vi "GetProbePlanCoordinates.vi"(8 "Use index as X coord":bool=TRUE, 9 "Probe Card Channels":i32=1) -> (0 "file path":string, 2 "OK?":bool, 3 "Array":T1(array[cluster]))   [LabVIEW 2018] (continued)
863\tX=17755.26\ty=25056.33 \nLabel=Strip\t864\tX=18099.17\ty=25163.49 \nLabel=Strip\t865\tX=17745.54\ty=25211.79 \nLabel=Strip\t866\tX=18089.41\ty=25319.09 \nLabel=Strip\t867\tX=17735.76\ty=25367.26 \nLabel=Strip\t868\tX=18079.58\ty=25474.68 \nLabel=Strip\t869\tX=17725.92\ty=25522.72 \nLabel=Strip\t870\tX=18069.70\ty=25630.28 \nLabel=Strip\t871\tX=17716.01\ty=25678.17 \nLabel=Strip\t872\tX=18059.75\ty=25785.87 \nLabel=Strip\t873\tX=17706.05\ty=25833.63 \nLabel=Strip\t874\tX=18049.75\ty=25941.46 \nLabel=Strip\t875\tX=17696.03\ty=25989.08 \nLabel=Strip\t876\tX=18039.68\ty=26097.04 \nLabel=Strip\t877\tX=17685.94\ty=26144.53 \nLabel=Strip\t878\tX=18029.56\ty=26252.63 \nLabel=Strip\t879\tX=17675.80\ty=26299.98 \nLabel=Strip\t880\tX=18019.37\ty=26408.21 \nLabel=Strip\t881\tX=17665.59\ty=26455.42 \nLabel=Strip\t882\tX=18009.13\ty=26563.79 \nLabel=Strip\t883\tX=17655.33\ty=26610.87 \nLabel=Strip\t884\tX=17998.82\ty=26719.39 \nLabel=Strip\t885\tX=17645.01\ty=26766.31 \nLabel=Strip\t886\tX=17988.45\ty=26874.93 \nLabel=Strip\t887\tX=17634.62\ty=26921.74 \nLabel=Strip\t888\tX=17978.03\ty=27030.50 \nLabel=Strip\t889\tX=17624.18\ty=27077.18 \nLabel=Strip\t890\tX=17967.54\ty=27186.07 \nLabel=Strip\t891\tX=17613.67\ty=27232.61 \nLabel=Strip\t892\tX=17956.99\ty=27341.64 \nLabel=Strip\t893\tX=17603.11\ty=27388.04 \nLabel=Strip\t894\tX=17946.37\ty=27497.34 \nLabel=Strip\t895\tX=17592.48\ty=27543.46 \nLabel=Strip\t896\tX=17935.72\ty=27652.76 \nLabel=Strip\t897\tX=17581.80\ty=27698.89 \nLabel=Strip\t898\tX=17924.99\ty=27808.31 \nLabel=Strip\t899\tX=17571.05\ty=27854.31 \nLabel=Strip\t900\tX=17914.20\ty=27963.87 \nLabel=Strip\t901\tX=17560.24\ty=28009.72 \nLabel=Strip\t902\tX=17903.35\ty=28119.42 \nLabel=Strip\t903\tX=17549.38\ty=28165.14 \nLabel=Strip\t904\tX=17892.45\ty=28274.96 \nLabel=Strip\t905\tX=17538.45\ty=28320.55 \nLabel=Strip\t906\tX=17881.48\ty=28430.51 \nLabel=Strip\t907\tX=17527.46\ty=28475.96 \nLabel=Strip\t908\tX=17870.45\ty=28586.05 \nLabel=Strip\t909\tX=17516.42\ty=28631.36 \nLabel=Strip\t910\tX=17859.36\ty=28741.59 \nLabel=Strip\t911\tX=17505.31\ty=28786.77 \nLabel=Strip\t912\tX=17848.21\ty=28897.13 \nLabel=Strip\t913\tX=17494.14\ty=28942.17 \nLabel=Strip\t914\tX=17837.00\ty=29052.66 \nLabel=Strip\t915\tX=17482.92\ty=29097.56 \nLabel=Strip\t916\tX=17825.73\ty=29208.19 \nLabel=Strip\t917\tX=17471.63\ty=29252.96 \nLabel=Strip\t918\tX=17814.40\ty=29363.71 \nLabel=Strip\t919\tX=17460.28\ty=29408.35 \nLabel=Strip\t920\tX=17803.00\ty=29519.24 \nLabel=Strip\t921\tX=17448.87\ty=29563.73 \nLabel=Strip\t922\tX=17791.55\ty=29674.76 \nLabel=Strip\t923\tX=17437.40\ty=29719.12 \nLabel=Strip\t924\tX=17780.04\ty=29830.28 \nLabel=Strip\t925\tX=17425.87\ty=29874.50 \nLabel=Strip\t926\tX=17768.47\ty=29985.79 \nLabel=Strip\t927\tX=17414.28\ty=30029.88 \nLabel=Strip\t928\tX=17756.84\ty=30141.30 \nLabel=Strip\t929\tX=17402.63\ty=30185.25 \nLabel=Strip\t930\tX=17745.15\ty=30296.81 \nLabel=Strip\t931\tX=17390.93\ty=30340.62 \nLabel=Strip\t932\tX=17733.39\ty=30452.31 \nLabel=Strip\t933\tX=17379.16\ty=30495.99 \nLabel=Strip\t934\tX=17721.58\ty=30607.81 \nLabel=Strip\t935\tX=17367.33\ty=30651.36 \nLabel=Strip\t936\tX=17709.71\ty=30763.31 \nLabel=Strip\t937\tX=17355.44\ty=30806.72 \nLabel=Strip\t938\tX=17697.77\ty=30918.81 \nLabel=Strip\t939\tX=17343.49\ty=30962.08 \nLabel=Strip\t940\tX=17685.78\ty=31074.30 \nLabel=Strip\t941\tX=17331.48\ty=31117.43 \nLabel=Strip\t942\tX=17673.73\ty=31229.79 \nLabel=Strip\t943\tX=17319.41\ty=31272.78 \nLabel=Strip\t944\tX=17661.61\ty=31385.27 \nLabel=Strip\t945\tX=17307.27\ty=31428.13 \nLabel=Strip\t946\tX=17649.44\ty=31540.75 \nLabel=Strip\t947\tX=17295.08\ty=31583.48 \nLabel=Strip\t948\tX=17637.20\ty=31696.23 \nLabel=Strip\t949\tX=17282.83\ty=31738.82 \nLabel=Strip\t950\tX=17624.91\ty=31851.70 \nLabel=Strip\t951\tX=17270.52\ty=31894.16 \nLabel=Strip\t952\tX=17612.55\ty=32007.17 \nLabel=Strip\t953\tX=17258.15\ty=32049.49 \nLabel=Strip\t954\tX=17600.14\ty=32162.64 \nLabel=Strip\t955\tX=17245.72\ty=32204.82 \nLabel=Strip\t956\tX=17587.66\ty=32318.10 \nLabel=Strip\t957\tX=17233.22\ty=32360.15 \nLabel=Strip\t958\tX=17575.13\ty=32473.56 \nLabel=Strip\t959\tX=17220.67\ty=32515.47 \nLabel=Strip\t960\tX=17562.53\ty=32629.02 \nLabel=Strip\t961\tX=17208.06\ty=32670.79 \nLabel=Strip\t962\tX=17549.87\ty=32784.47 \nLabel=Strip\t963\tX=17195.39\ty=32826.11 \nLabel=Strip\t964\tX=17537.16\ty=32939.92 \nLabel=Strip\t965\tX=17182.65\ty=32981.42 \nLabel=Strip\t966\tX=17524.38\ty=33095.37 \nLabel=Strip\t967\tX=17169.86\ty=33136.73 \nLabel=Strip\t968\tX=17511.54\ty=33250.81 \nLabel=Strip\t969\tX=17157.01\ty=33292.04 \nLabel=Strip\t970\tX=17498.64\ty=33406.25 \nLabel=Strip\t971\tX=17144.09\ty=33447.34 \nLabel=Strip\t972\tX=17485.69\ty=33561.68 \nLabel=Strip\t973\tX=17131.12\ty=33602.64 \nLabel=Strip\t974\tX=17472.67\ty=33717.12 \nLabel=Strip\t975\tX=17118.09\ty=33757.93 \nLabel=Strip\t976\tX=17459.59\ty=33872.54 \nLabel=Strip\t977\tX=17104.99\ty=33913.23 \nLabel=Strip\t978\tX=17446.45\ty=34027.97 \nLabel=Strip\t979\tX=17091.84\ty=34068.51 \nLabel=Strip\t980\tX=17433.25\ty=34183.39 \nLabel=Strip\t981\tX=17078.62\ty=34223.80 \nLabel=Strip\t982\tX=17419.99\ty=34338.80 \nLabel=Strip\t983\tX=17065.35\ty=34379.08 \nLabel=Strip\t984\tX=17406.67\ty=34494.21 \nLabel=Strip\t985\tX=17052.01\ty=34534.35 \nLabel=Strip\t986\tX=17393.29\ty=34649.62 \nLabel=Strip\t987\tX=17038.62\ty=34689.62 \nLabel=Strip\t988\tX=17379.85\ty=34805.03 \nLabel=Strip\t989\tX=17025.16\ty=34844.89 \nLabel=Strip\t990\tX=17366.35\ty=34960.43 \nLabel=Strip\t991\tX=17011.65\ty=35000.16 \nLabel=Strip\t992\tX=17352.79\ty=35115.82 \nLabel=Strip\t993\tX=16998.07\ty=35155.42 \nLabel=Strip\t994\tX=17339.17\ty=35271.21 \nLabel=Strip\t995\tX=16984.43\ty=35310.67 \nLabel=Strip\t996\tX=17325.49\ty=35426.60 \nLabel=Strip\t997\tX=16970.74\ty=35465.92 \nLabel=Strip\t998\tX=17311.75\ty=35581.99 \nLabel=Strip\t999\tX=16956.98\ty=35621.17 \nLabel=Strip\t1000\tX=17297.95\ty=35737.37 \nLabel=Strip\t1001\tX=16943.16\ty=35776.42 \nLabel=Strip\t1002\tX=17284.09\ty=35892.74 \nLabel=Strip\t1003\tX=16929.29\ty=35931.66 \nLabel=Strip\t1004\tX=17270.17\ty=36048.12 \nLabel=Strip\t1005\tX=16915.35\ty=36086.89 \nLabel=Strip\t1006\tX=17256.18\ty=36203.49 \nLabel=Strip\t1007\tX=16901.35\ty=36242.12 \nLabel=Strip\t1008\tX=17242.14\ty=36358.85 \nLabel=Strip\t1009\tX=16887.30\ty=36397.35 \nLabel=Strip\t1010\tX=17228.04\ty=36514.21 \nLabel=Strip\t1011\tX=16873.18\ty=36552.57 \nLabel=Strip\t1012\tX=17213.87\ty=36669.56 \nLabel=Strip\t1013\tX=16859.00\ty=36707.79 \nLabel=Strip\t1014\tX=17199.65\ty=36824.92 \nLabel=Strip\t1015\tX=16844.76\ty=36863.01 \nLabel=Strip\t1016\tX=17185.37\ty=36980.26 \nLabel=Strip\t1017\tX=16830.46\ty=37018.22 \nLabel=Strip\t1018\tX=17171.03\ty=37135.61 \nLabel=Strip\t1019\tX=16816.11\ty=37173.43 \nLabel=Strip\t1020\tX=17156.62\ty=37290.95 \nLabel=Strip\t1021\tX=16801.69\ty=37328.63 \nLabel=Strip\t1022\tX=17142.16\ty=37446.28 \nLabel=Strip\t1023\tX=16787.21\ty=37483.83 \nLabel=Strip\t1024\tX=17127.63\ty=37601.61 \nLabel=Strip\t1025\tX=16772.67\ty=37639.02 \nLabel=Strip\t1026\tX=17113.05\ty=37756.94 \nRegion=Segment\t2B\nLabel=Strip\t1\tX=17590.21\ty=-41968.68 \nLabel=Strip\t2\tX=17947.11\ty=-41920.02 \nLabel=Strip\t3\tX=17606.36\ty=-41813.84 \nLabel=Strip\t4\tX=17963.24\ty=-41765.04 \nLabel=Strip\t5\tX=17622.45\ty=-41658.99 \nLabel=Strip\t6\tX=17979.31\ty=-41610.05 \nLabel=Strip\t7\tX=17638.47\ty=-41504.13 \nLabel=Strip\t8\tX=17995.31\ty=-41455.05 \nLabel=Strip\t9\tX=17654.44\ty=-41349.26 \nLabel=Strip\t10\tX=18011.26\ty=-41300.04 \nLabel=Strip\t11\tX=17670.35\ty=-41194.38 \nLabel=Strip\t12\tX=18027.15\ty=-41145.03 \nLabel=Strip\t13\tX=17686.20\ty=-41039.50 \nLabel=Strip\t14\tX=18042.98\ty=-40990.01 \nLabel=Strip\t15\tX=17701.99\ty=-40884.61 \nLabel=Strip\t16\tX=18058.75\ty=-40834.98 \nLabel=Strip\t17\tX=17717.72\ty=-40729.71 \nLabel=Strip\t18\tX=18074.46\ty=-40679.94 \nLabel=Strip\t19\tX=17733.38\ty=-40574.81 \nLabel=Strip\t20\tX=18090.11\ty=-40524.90 \nLabel=Strip\t21\tX=17748.99\ty=-40419.89 \nLabel=Strip\t22\tX=18105.70\ty=-40369.85 \nLabel=Strip\t23\tX=17764.54\ty=-40264.98 \nLabel=Strip\t24\tX=18121.23\ty=-40214.79 \nLabel=Strip\t25\tX=17780.04\ty=-40110.05 \nLabel=Strip\t26\tX=18136.71\ty=-40059.73 \nLabel=Strip\t27\tX=17795.47\ty=-39955.11 \nLabel=Strip\t28\tX=18152.12\ty=-39904.65 \nLabel=Strip\t29\tX=17810.84\ty=-39800.17 \nLabel=Strip\t30\tX=18167.47\ty=-39749.57 \nLabel=Strip\t31\tX=17826.15\ty=-39645.22 \nLabel=Strip\t32\tX=18182.76\ty=-39594.49 \nLabel=Strip\t33\tX=17841.40\ty=-39490.27 \nLabel=Strip\t34\tX=18197.99\ty=-39439.39 \nLabel=Strip\t35\tX=17856.60\ty=-39335.31 \nLabel=Strip\t36\tX=18213.17\ty=-39284.29 \nLabel=Strip\t37\tX=17871.73\ty=-39180.34 \nLabel=Strip\t38\tX=18228.28\ty=-39129.18 \nLabel=Strip\t39\tX=17886.80\ty=-39025.36 \nLabel=Strip\t40\tX=18243.34\ty=-38974.07 \nLabel=Strip\t41\tX=17901.82\ty=-38870.38 \nLabel=Strip\t42\tX=18258.33\ty=-38818.95 \nLabel=Strip\t43\tX=17916.77\ty=-38715.38 \nLabel=Strip\t44\tX=18273.27\ty=-38663.82 \nLabel=Strip\t45\tX=17931.67\ty=-38560.39 \nLabel=Strip\t46\tX=18288.14\ty=-38508.68 \nLabel=Strip\t47\tX=17946.50\ty=-38405.38 \nLabel=Strip\t48\tX=18302.96\ty=-38353.54 \nLabel=Strip\t49\tX=17961.28\ty=-38250.37 \nLabel=Strip\t50\tX=18317.71\ty=-38198.39 \nLabel=Strip\t51\tX=17975.99\ty=-38095.35 \nLabel=Strip\t52\tX=18332.41\ty=-38043.23 \nLabel=Strip\t53\tX=17990.65\ty=-37940.32 \nLabel=Strip\t54\tX=18347.04\ty=-37888.06 \nLabel=Strip\t55\tX=18005.25\ty=-37785.29 \nLabel=Strip\t56\tX=18361.62\ty=-37732.89 \nLabel=Strip\t57\tX=18019.78\ty=-37630.25 \nLabel=Strip\t58\tX=18376.14\ty=-37577.71 \nLabel=Strip\t59\tX=18034.26\ty=-37475.20 \nLabel=Strip\t60\tX=18390.59\ty=-37422.53 \nLabel=Strip\t61\tX=18048.68\ty=-37320.15 \nLabel=Strip\t62\tX=18404.99\ty=-37267.34 \nLabel=Strip\t63\tX=18063.04\ty=-37165.09 \nLabel=Strip\t64\tX=18419.33\ty=-37112.14 \nLabel=Strip\t65\tX=18077.33\ty=-37010.02 \nLabel=Strip\t66\tX=18433.61\ty=-36956.93 \nLabel=Strip\t67\tX=18091.57\ty=-36854.95 \nLabel=Strip\t68\tX=18447.83\ty=-36801.72 \nLabel=Strip\t69\tX=18105.75\ty=-36699.86 \nLabel=Strip\t70\tX=18461.98\ty=-36646.50 \nLabel=Strip\t71\tX=18119.87\ty=-36544.78 \nLabel=Strip\t72\tX=18476.08\ty=-36491.27 \nLabel=Strip\t73\tX=18133.93\ty=-36389.68 \nLabel=Strip\t74\tX=18490.12\ty=-36336.04 \nLabel=Strip\t75\tX=18147.93\ty=-36234.58 \nLabel=Strip\t76\tX=18504.10\ty=-36180.80 \nLabel=Strip\t77\tX=18161.87\ty=-36079.47 \nLabel=Strip\t78\tX=18518.02\ty=-36025.55 \nLabel=Strip\t79\tX=18175.75\ty=-35924.36 \nLabel=Strip\t80\tX=18531.88\ty=-35870.30 \nLabel=Strip\t81\tX=18189.57\ty=-35769.24 \nLabel=Strip\t82\tX=18545.68\ty=-35715.04 \nLabel=Strip\t83\tX=18203.33\ty=-35614.11 \nLabel=Strip\t84\tX=18559.42\ty=-35559.78 \nLabel=Strip\t85\tX=18217.04\ty=-35458.97 \nLabel=Strip\t86\tX=18573.10\ty=-35404.50 \nLabel=Strip\t87\tX=18230.68\ty=-35303.83 \nLabel=Strip\t88\tX=18586.72\ty=-35249.22 \nLabel=Strip\t89\tX=18244.26\ty=-35148.69 \nLabel=Strip\t90\tX=18600.28\ty=-35093.94 \nLabel=Strip\t91\tX=18257.78\ty=-34993.53 \nLabel=Strip\t92\tX=18613.78\ty=-34938.65 \nLabel=Strip\t93\tX=18271.25\ty=-34838.37 \nLabel=Strip\t94\tX=18627.23\ty=-34783.35 \nLabel=Strip\t95\tX=18284.65\ty=-34683.20 \nLabel=Strip\t96\tX=18640.61\ty=-34628.04 \nLabel=Strip\t97\tX=18297.99\ty=-34528.03 \nLabel=Strip\t98\tX=18653.93\ty=-34472.73 \nLabel=Strip\t99\tX=18311.28\ty=-34372.85 \nLabel=Strip\t100\tX=18667.19\ty=-34317.41 \nLabel=Strip\t101\tX=18324.50\ty=-34217.66 \nLabel=Strip\t102\tX=18680.40\ty=-34162.09 \nLabel=Strip\t103\tX=18337.66\ty=-34062.47 \nLabel=Strip\t104\tX=18693.54\ty=-34006.76 \nLabel=Strip\t105\tX=18350.77\ty=-33907.27 \nLabel=Strip\t106\tX=18706.62\ty=-33851.42 \nLabel=Strip\t107\tX=18363.81\ty=-33752.06 \nLabel=Strip\t108\tX=18719.64\ty=-33696.08 \nLabel=Strip\t109\tX=18376.80\ty=-33596.85 \nLabel=Strip\t110\tX=18732.61\ty=-33540.73 \nLabel=Strip\t111\tX=18389.72\ty=-33441.64 \nLabel=Strip\t112\tX=18745.51\ty=-33385.37 \nLabel=Strip\t113\tX=18402.59\ty=-33286.41 \nLabel=Strip\t114\tX=18758.35\ty=-33230.01 \nLabel=Strip\t115\tX=18415.39\ty=-33131.18 \nLabel=Strip\t116\tX=18771.14\ty=-33074.64 \nLabel=Strip\t117\tX=18428.14\ty=-32975.94 \nLabel=Strip\t118\tX=18783.86\ty=-32919.26 \nLabel=Strip\t119\tX=18440.83\ty=-32820.70 \nLabel=Strip\t120\tX=18796.53\ty=-32763.88 \nLabel=Strip\t121\tX=18453.45\ty=-32665.45 \nLabel=Strip\t122\tX=18809.13\ty=-32608.49 \nLabel=Strip\t123\tX=18466.02\ty=-32510.19 \nLabel=Strip\t124\tX=18821.68\ty=-32453.10 \nLabel=Strip\t125\tX=18478.53\ty=-32354.93 \nLabel=Strip\t126\tX=18834.16\ty=-32297.70 \nLabel=Strip\t127\tX=18490.97\ty=-32199.67 \nLabel=Strip\t128\tX=18846.59\ty=-32142.30 \nLabel=Strip\t129\tX=18503.36\ty=-32044.39 \nLabel=Strip\t130\tX=18858.95\ty=-31986.88 \nLabel=Strip\t131\tX=18515.69\ty=-31889.11 \nLabel=Strip\t132\tX=18871.26\ty=-31831.47 \nLabel=Strip\t133\tX=18527.96\ty=-31733.83 \nLabel=Strip\t134\tX=18883.50\ty=-31676.04 \nLabel=Strip\t135\tX=18540.16\ty=-31578.53 \nLabel=Strip\t136\tX=18895.69\ty=-31520.61 \nLabel=Strip\t137\tX=18552.31\ty=-31423.24 \nLabel=Strip\t138\tX=18907.81\ty=-31365.18 \nLabel=Strip\t139\tX=18564.40\ty=-31267.93 \nLabel=Strip\t140\tX=18919.88\ty=-31209.73 \nLabel=Strip\t141\tX=18576.43\ty=-31112.62 \nLabel=Strip\t142\tX=18931.89\ty=-31054.29 \nLabel=Strip\t143\tX=18588.40\ty=-30957.31 \nLabel=Strip\t144\tX=18943.83\ty=-30898.83 \nLabel=Strip\t145\tX=18600.31\ty=-30801.99 \nLabel=Strip\t146\tX=18955.72\ty=-30743.37 \nLabel=Strip\t147\tX=18612.16\ty=-30646.66 \nLabel=Strip\t148\tX=18967.55\ty=-30587.91 \nLabel=Strip\t149\tX=18623.94\ty=-30491.32 \nLabel=Strip\t150\tX=18979.31\ty=-30432.44 \nLabel=Strip\t151\tX=18635.67\ty=-30335.98 \nLabel=Strip\t152\tX=18991.02\ty=-30276.96 \nLabel=Strip\t153\tX=18647.34\ty=-30180.64 \nLabel=Strip\t154\tX=19002.67\ty=-30121.48 \nLabel=Strip\t155\tX=18658.95\ty=-30025.29 \nLabel=Strip\t156\tX=19014.25\ty=-29965.99 \nLabel=Strip\t157\tX=18670.50\ty=-29869.93 \nLabel=Strip\t158\tX=19025.78\ty=-29810.49 \nLabel=Strip\t159\tX=18682.00\ty=-29714.57 \nLabel=Strip\t160\tX=19037.25\ty=-29654.99 \nLabel=Strip\t161\tX=18693.43\ty=-29559.20 \nLabel=Strip\t162\tX=19048.66\ty=-29499.49 \nLabel=Strip\t163\tX=18704.80\ty=-29403.83 \nLabel=Strip\t164\tX=19060.00\ty=-29343.98 \nLabel=Strip\t165\tX=18716.11\ty=-29248.45 \nLabel=Strip\t166\tX=19071.29\ty=-29188.46 \nLabel=Strip\t167\tX=18727.36\ty=-29093.06 \nLabel=Strip\t168\tX=19082.52\ty=-29032.93 \nLabel=Strip\t169\tX=18738.55\ty=-28937.67 \nLabel=Strip\t170\tX=19093.69\ty=-28877.41 \nLabel=Strip\t171\tX=18749.68\ty=-28782.28 \nLabel=Strip\t172\tX=19104.80\ty=-28721.87 \nLabel=Strip\t173\tX=18760.75\ty=-28626.87 \nLabel=Strip\t174\tX=19115.84\ty=-28566.33 \nLabel=Strip\t175\tX=18771.76\ty=-28471.47 \nLabel=Strip\t176\tX=19126.83\ty=-28410.79 \nLabel=Strip\t177\tX=18782.72\ty=-28316.05 \nLabel=Strip\t178\tX=19137.76\ty=-28255.24 \nLabel=Strip\t179\tX=18793.61\ty=-28160.63 \nLabel=Strip\t180\tX=19148.63\ty=-28099.68 \nLabel=Strip\t181\tX=18804.44\ty=-28005.21 \nLabel=Strip\t182\tX=19159.44\ty=-27944.12 \nLabel=Strip\t183\tX=18815.21\ty=-27849.78 \nLabel=Strip\t184\tX=19170.19\ty=-27788.55 \nLabel=Strip\t185\tX=18825.92\ty=-27694.35 \nLabel=Strip\t186\tX=19180.88\ty=-27632.98 \nLabel=Strip\t187\tX=18836.58\ty=-27538.90 \nLabel=Strip\t188\tX=19191.50\ty=-27477.40 \nLabel=Strip\t189\tX=18847.17\ty=-27383.46 \nLabel=Strip\t190\tX=19202.07\ty=-27321.82 \nLabel=Strip\t191\tX=18857.70\ty=-27228.01 \nLabel=Strip\t192\tX=19212.58\ty=-27166.23 \nLabel=Strip\t193\tX=18868.17\ty=-27072.55 \nLabel=Strip\t194\tX=19223.03\ty=-27010.63 \nLabel=Strip\t195\tX=18878.59\ty=-26917.09 \nLabel=Strip\t196\tX=19233.42\ty=-26855.03 \nLabel=Strip\t197\tX=18888.94\ty=-26761.62 \nLabel=Strip\t198\tX=19243.75\ty=-26699.43 \nLabel=Strip\t199\tX=18899.23\ty=-26606.15 \nLabel=Strip\t200\tX=19254.02\ty=-26543.82 \nLabel=Strip\t201\tX=18909.47\ty=-26450.67 \nLabel=Strip\t202\tX=19264.23\ty=-26388.20 \nLabel=Strip\t203\tX=18919.64\ty=-26295.19 \nLabel=Strip\t204\tX=19274.38\ty=-26232.58 \nLabel=Strip\t205\tX=18929.75\ty=-26139.70 \nLabel=Strip\t206\tX=19284.47\ty=-26076.96 \nLabel=Strip\t207\tX=18939.81\ty=-25984.21 \nLabel=Strip\t208\tX=19294.50\ty=-25921.32 \nLabel=Strip\t209\tX=18949.80\ty=-25828.71 \nLabel=Strip\t210\tX=19304.47\ty=-25765.69 \nLabel=Strip\t211\tX=18959.74\ty=-25673.20 \nLabel=Strip\t212\tX=19314.38\ty=-25610.05 \nLabel=Strip\t213\tX=18969.61\ty=-25517.70 \nLabel=Strip\t214\tX=19324.23\ty=-25454.40 \nLabel=Strip\t215\tX=18979.42\ty=-25362.18 \nLabel=Strip\t216\tX=19334.02\ty=-25298.75 \nLabel=Strip\t217\tX=18989.18\ty=-25206.66 \nLabel=Strip\t218\tX=19343.74\ty=-25143.09 \nLabel=Strip\t219\tX=18998.87\ty=-25051.14 \nLabel=Strip\t220\tX=19353.41\ty=-24987.43 \nLabel=Strip\t221\tX=19008.51\ty=-24895.61 \nLabel=Strip\t222\tX=19363.02\ty=-24831.76 \nLabel=Strip\t223\tX=19018.08\ty=-24740.08 \nLabel=Strip\t224\tX=19372.57\ty=-24676.09 \nLabel=Strip\t225\tX=19027.60\ty=-24584.54 \nLabel=Strip\t226\tX=19382.06\ty=-24520.42 \nLabel=Strip\t227\tX=19037.05\ty=-24428.99 \nLabel=Strip\t228\tX=19391.49\ty=-24364.73 \nLabel=Strip\t229\tX=19046.44\ty=-24273.44 \nLabel=Strip\t230\tX=19400.86\ty=-24209.05 \nLabel=Strip\t231\tX=19055.78\ty=-24117.89 \nLabel=Strip\t232\tX=19410.17\ty=-24053.36 \nLabel=Strip\t233\tX=19065.05\ty=-23962.33 \nLabel=Strip\t234\tX=19419.42\ty=-23897.66 \nLabel=Strip\t235\tX=19074.27\ty=-23806.77 \nLabel=Strip\t236\tX=19428.61\ty=-23741.96 \nLabel=Strip\t237\tX=19083.42\ty=-23651.20 \nLabel=Strip\t238\tX=19437.74\ty=-23586.25 \nLabel=Strip\t239\tX=19092.52\ty=-23495.63 \nLabel=Strip\t240\tX=19446.81\ty=-23430.54 \nLabel=Strip\t241\tX=19101.55\ty=-23340.05 \nLabel=Strip\t242\tX=19455.82\ty=-23274.83 \nLabel=Strip\t243\tX=19110.53\ty=-23184.46 \nLabel=Strip\t244\tX=19464.77\ty=-23119.11 \nLabel=Strip\t245\tX=19119.44\ty=-23028.88 \nLabel=Strip\t246\tX=19473.66\ty=-22963.38 \nLabel=Strip\t247\tX=19128.30\ty=-22873.28 \nLabel=Strip\t248\tX=19482.49\ty=-22807.63 \nLabel=Strip\t249\tX=19137.09\ty=-22717.69 \nLabel=Strip\t250\tX=19491.26\ty=-22651.92 \nLabel=Strip\t251\tX=19145.83\ty=-22562.08 \nLabel=Strip\t252\tX=19499.97\ty=-22496.18 \nLabel=Strip\t253\tX=19154.50\ty=-22406.48 \nLabel=Strip\t254\tX=19508.62\ty=-22340.43 \nLabel=Strip\t255\tX=19163.12\ty=-22250.87 \nLabel=Strip\t256\tX=19517.21\ty=-22184.68 \nLabel=Strip\t257\tX=19171.67\ty=-22095.25 \nLabel=Strip\t258\tX=19525.74\ty=-22028.93 \nLabel=Strip\t259\tX=19180.17\ty=-21939.63 \nLabel=Strip\t260\tX=19534.21\ty=-21873.17 \nLabel=Strip\t261\tX=19188.60\ty=-21784.01 \nLabel=Strip\t262\tX=19542.62\ty=-21717.41 \nLabel=Strip\t263\tX=19196.98\ty=-21628.38 \nLabel=Strip\t264\tX=19550.97\ty=-21561.64 \nLabel=Strip\t265\tX=19205.30\ty=-21472.74 \nLabel=Strip\t266\tX=19559.26\ty=-21405.87 \nLabel=Strip\t267\tX=19213.55\ty=-21317.10 \nLabel=Strip\t268\tX=19567.49\ty=-21250.10 \nLabel=Strip\t269\tX=19221.75\ty=-21161.46 \nLabel=Strip\t270\tX=19575.66\ty=-21094.32 \nLabel=Strip\t271\tX=19229.88\ty=-21005.81 \nLabel=Strip\t272\tX=19583.77\ty=-20938.53 \nLabel=Strip\t273\tX=19237.96\ty=-20850.16 \nLabel=Strip\t274\tX=19591.82\ty=-20782.74 \nLabel=Strip\t275\tX=19245.97\ty=-20694.50 \nLabel=Strip\t276\tX=19599.81\ty=-20626.95 \nLabel=Strip\t277\tX=19253.93\ty=-20538.84 \nLabel=Strip\t278\tX=19607.74\ty=-20471.15 \nLabel=Strip\t279\tX=19261.82\ty=-20383.18 \nLabel=Strip\t280\tX=19615.61\ty=-20315.35 \nLabel=Strip\t281\tX=19269.66\ty=-20227.51 \nLabel=Strip\t282\tX=19623.42\ty=-20159.54 \nLabel=Strip\t283\tX=19277.43\ty=-20071.84 \nLabel=Strip\t284\tX=19631.16\ty=-20003.73 \nLabel=Strip\t285\tX=19285.15\ty=-19916.16 \nLabel=Strip\t286\tX=19638.85\ty=-19847.92 \nLabel=Strip\t287\tX=19292.81\ty=-19760.48 \nLabel=Strip\t288\tX=19646.48\ty=-19692.10 \nLabel=Strip\t289\tX=19300.40\ty=-19604.79 \nLabel=Strip\t290\tX=19654.05\ty=-19536.27 \nLabel=Strip\t291\tX=19307.94\ty=-19449.10 \nLabel=Strip\t292\tX=19661.56\ty=-19380.44 \nLabel=Strip\t293\tX=19315.41\ty=-19293.40 \nLabel=Strip\t294\tX=19669.01\ty=-19224.61 \nLabel=Strip\t295\tX=19322.83\ty=-19137.70 \nLabel=Strip\t296\tX=19676.40\ty=-19068.78 \nLabel=Strip\t297\tX=19330.18\ty=-18982.00 \nLabel=Strip\t298\tX=19683.73\ty=-18912.94 \nLabel=Strip\t299\tX=19337.48\ty=-18826.29 \nLabel=Strip\t300\tX=19691.00\ty=-18757.09 \nLabel=Strip\t301\tX=19344.71\ty=-18670.58 \nLabel=Strip\t302\tX=19698.20\ty=-18601.24 \nLabel=Strip\t303\tX=19351.89\ty=-18514.87 \nLabel=Strip\t304\tX=19705.35\ty=-18445.39 \nLabel=Strip\t305\tX=19359.00\ty=-18359.15 \nLabel=Strip\t306\tX=19712.44\ty=-18289.53 \nLabel=Strip\t307\tX=19366.06\ty=-18203.42 \nLabel=Strip\t308\tX=19719.47\ty=-18133.67 \nLabel=Strip\t309\tX=19373.05\ty=-18047.70 \nLabel=Strip\t310\tX=19726.44\ty=-17977.81 \nLabel=Strip\t311\tX=19379.99\ty=-17891.96 \nLabel=Strip\t312\tX=19733.35\ty=-17821.94 \nLabel=Strip\t313\tX=19386.86\ty=-17736.23 \nLabel=Strip\t314\tX=19740.19\ty=-17666.06 \nLabel=Strip\t315\tX=19393.68\ty=-17580.49 \nLabel=Strip\t316\tX=19746.98\ty=-17510.19 \nLabel=Strip\t317\tX=19400.43\ty=-17424.74 \nLabel=Strip\t318\tX=19753.71\ty=-17354.31 \nLabel=Strip\t319\tX=19407.13\ty=-17269.00 \nLabel=Strip\t320\tX=19760.38\ty=-17198.42 \nLabel=Strip\t321\tX=19413.76\ty=-17113.25 \nLabel=Strip\t322\tX=19766.98\ty=-17042.53 \nLabel=Strip\t323\tX=19420.34\ty=-16957.49 \nLabel=Strip\t324\tX=19773.53\ty=-16886.64 \nLabel=Strip\t325\tX=19426.85\ty=-16801.73 \nLabel=Strip\t326\tX=19780.02\ty=-16730.75 \nLabel=Strip\t327\tX=19433.31\ty=-16645.97 \nLabel=Strip\t328\tX=19786.45\ty=-16574.85 \nLabel=Strip\t329\tX=19439.70\ty=-16490.20 \nLabel=Strip\t330\tX=19792.81\ty=-16418.94 \nLabel=Strip\t331\tX=19446.04\ty=-16334.43 \nLabel=Strip\t332\tX=19799.12\ty=-16263.04 \nLabel=Strip\t333\tX=19452.31\ty=-16178.66 \nLabel=Strip\t334\tX=19805.37\ty=-16107.12 \nLabel=Strip\t335\tX=19458.53\ty=-16022.88 \nLabel=Strip\t336\tX=19811.55\ty=-15951.21 \nLabel=Strip\t337\tX=19464.68\ty=-15867.10 \nLabel=Strip\t338\tX=19817.68\ty=-15795.29 \nLabel=Strip\t339\tX=19470.77\ty=-15711.31 \nLabel=Strip\t340\tX=19823.75\ty=-15639.37 \nLabel=Strip\t341\tX=19476.81\ty=-15555.52 \nLabel=Strip\t342\tX=19829.75\ty=-15483.44 \nLabel=Strip\t343\tX=19482.78\ty=-15399.73 \nLabel=Strip\t344\tX=19835.70\ty=-15327.51 \nLabel=Strip\t345\tX=19488.70\ty=-15243.93 \nLabel=Strip\t346\tX=19841.59\ty=-15171.58 \nLabel=Strip\t347\tX=19494.55\ty=-15088.13 \nLabel=Strip\t348\tX=19847.41\ty=-15015.64 \nLabel=Strip\t349\tX=19500.34\ty=-14932.33 \nLabel=Strip\t350\tX=19853.18\ty=-14859.70 \nLabel=Strip\t351\tX=19506.08\ty=-14776.53 \nLabel=Strip\t352\tX=19858.88\ty=-14703.76 \nLabel=Strip\t353\tX=19511.75\ty=-14620.71 \nLabel=Strip\t354\tX=19864.53\ty=-14547.81 \nLabel=Strip\t355\tX=19517.36\ty=-14464.90 \nLabel=Strip\t356\tX=19870.11\ty=-14391.86 \nLabel=Strip\t357\tX=19522.92\ty=-14309.08 \nLabel=Strip\t358\tX=19875.64\ty=-14235.91 \nLabel=Strip\t359\tX=19528.41\ty=-14153.26 \nLabel=Strip\t360\tX=19881.11\ty=-14079.95 \nLabel=Strip\t361\tX=19533.84\ty=-13997.44 \nLabel=Strip\t362\tX=19886.51\ty=-13923.99 \nLabel=Strip\t363\tX=19539.22\ty=-13841.61 \nLabel=Strip\t364\tX=19891.85\ty=-13768.02 \nLabel=Strip\t365\tX=19544.53\ty=-13685.78 \nLabel=Strip\t366\tX=19897.14\ty=-13612.06 \nLabel=Strip\t367\tX=19549.78\ty=-13529.95 \nLabel=Strip\t368\tX=19902.36\ty=-13456.09 \nLabel=Strip\t369\tX=19554.98\ty=-13374.11 \nLabel=Strip\t370\tX=19907.53\ty=-13300.11 \nLabel=Strip\t371\tX=19560.11\ty=-13218.27 \nLabel=Strip\t372\tX=19912.63\ty=-13144.13 \nLabel=Strip\t373\tX=19565.18\ty=-13062.42 \nLabel=Strip\t374\tX=19917.68\ty=-12988.15 \nLabel=Strip\t375\tX=19570.19\ty=-12906.58 \nLabel=Strip\t376\tX=19922.66\ty=-12832.17 \nLabel=Strip\t377\tX=19575.15\ty=-12750.73 \nLabel=Strip\t378\tX=19927.58\ty=-12676.18 \nLabel=Strip\t379\tX=19580.04\ty=-12594.87 \nLabel=Strip\t380\tX=19932.45\ty=-12520.19 \nLabel=Strip\t381\tX=19584.87\ty=-12439.02 \nLabel=Strip\t382\tX=19937.25\ty=-12364.20 \nLabel=Strip\t383\tX=19589.64\ty=-12283.16 \nLabel=Strip\t384\tX=19941.99\ty=-12208.20 \nLabel=Strip\t385\tX=19594.35\ty=-12127.29 \nLabel=Strip\t386\tX=19946.68\ty=-12052.20 \nLabel=Strip\t387\tX=19599.01\ty=-11971.43 \nLabel=Strip\t388\tX=19951.30\ty=-11896.20 \nLabel=Strip\t389\tX=19603.60\ty=-11815.56 \nLabel=Strip\t390\tX=19955.86\ty=-11740.19 \nLabel=Strip\t391\tX=19608.13\ty=-11659.68 \nLabel=Strip\t392\tX=19960.36\ty=-11584.18 \nLabel=Strip\t393\tX=19612.60\ty=-11503.81 \nLabel=Strip\t394\tX=19964.81\ty=-11428.17 \nLabel=Strip\t395\tX=19617.01\ty=-11347.93 \nLabel=Strip\t396\tX=19969.19\ty=-11272.15 \nLabel=Strip\t397\tX=19621.36\ty=-11192.05 \nLabel=Strip\t398\tX=19973.51\ty=-11116.14 \nLabel=Strip\t399\tX=19625.65\ty=-11036.16 \nLabel=Strip\t400\tX=19977.77\ty=-10960.11 \nLabel=Strip\t401\tX=19629.88\ty=-10880.28 \nLabel=Strip\t402\tX=19981.97\ty=-10804.09 \nLabel=Strip\t403\tX=19634.05\ty=-10724.38 \nLabel=Strip\t404\tX=19986.11\ty=-10648.06 \nLabel=Strip\t405\tX=19638.17\ty=-10568.10 \nLabel=Strip\t406\tX=19990.20\ty=-10491.46 \nLabel=Strip\t407\tX=19642.22\ty=-10412.36 \nLabel=Strip\t408\tX=19994.22\ty=-10335.72 \nLabel=Strip\t409\tX=19646.21\ty=-10256.62 \nLabel=Strip\t410\tX=19998.18\ty=-10179.98 \nLabel=Strip\t411\tX=19650.14\ty=-10100.88 \nLabel=Strip\t412\tX=20002.07\ty=-10024.23 \nLabel=Strip\t413\tX=19654.00\ty=-9945.13 \nLabel=Strip\t414\tX=20005.91\ty=-9868.48 \nLabel=Strip\t415\tX=19657.81\ty=-9789.38 \nLabel=Strip\t416\tX=20009.70\ty=-9711.84 \nLabel=Strip\t417\tX=19661.56\ty=-9633.07 \nLabel=Strip\t418\tX=20013.42\ty=-9555.79 \nLabel=Strip\t419\tX=19665.25\ty=-9477.16 \nLabel=Strip\t420\tX=20017.08\ty=-9399.74 \nLabel=Strip\t421\tX=19668.88\ty=-9321.24 \nLabel=Strip\t422\tX=20020.67\ty=-9243.69 \nLabel=Strip\t423\tX=19672.45\ty=-9165.32 \nLabel=Strip\t424\tX=20024.21\ty=-9087.64 \nLabel=Strip\t425\tX=19675.96\ty=-9009.40 \nLabel=Strip\t426\tX=20027.69\ty=-8931.58 \nLabel=Strip\t427\tX=19679.41\ty=-8853.48 \nLabel=Strip\t428\tX=20031.11\ty=-8775.52 \nLabel=Strip\t429\tX=19682.80\ty=-8697.55 \nLabel=Strip\t430\tX=20034.47\ty=-8619.46 \nLabel=Strip\t431\tX=19686.13\ty=-8541.62 \nLabel=Strip\t432\tX=20037.77\ty=-8463.39 \nLabel=Strip\t433\tX=19689.39\ty=-8385.69 \nLabel=Strip\t434\tX=20041.00\ty=-8307.32 \nLabel=Strip\t435\tX=19692.60\ty=-8229.76 \nLabel=Strip\t436\tX=20044.18\ty=-8151.25 \nLabel=Strip\t437\tX=19695.75\ty=-8073.82 \nLabel=Strip\t438\tX=20047.30\ty=-7995.18 \nLabel=Strip\t439\tX=19698.84\ty=-7917.88 \nLabel=Strip\t440\tX=20050.36\ty=-7839.10 \nLabel=Strip\t441\tX=19701.86\ty=-7761.94 \nLabel=Strip\t442\tX=20053.35\ty=-7683.02 \nLabel=Strip\t443\tX=19704.83\ty=-7606.00 \nLabel=Strip\t444\tX=20056.29\ty=-7526.94 \nLabel=Strip\t445\tX=19707.74\ty=-7450.05 \nLabel=Strip\t446\tX=20059.17\ty=-7370.86 \nLabel=Strip\t447\tX=19710.58\ty=-7294.10 \nLabel=Strip\t448\tX=20061.98\ty=-7214.78 \nLabel=Strip\t449\tX=19713.37\ty=-7138.15 \nLabel=Strip\t450\tX=20064.74\ty=-7058.69 \nLabel=Strip\t451\tX=19716.10\ty=-6982.19 \nLabel=Strip\t452\tX=20067.43\ty=-6902.60 \nLabel=Strip\t453\tX=19718.76\ty=-6826.24 \nLabel=Strip\t454\tX=20070.07\ty=-6746.51 \nLabel=Strip\t455\tX=19721.37\ty=-6670.28 \nLabel=Strip\t456\tX=20072.65\ty=-6590.41 \nLabel=Strip\t457\tX=19723.92\ty=-6514.32 \nLabel=Strip\t458\tX=20075.16\ty=-6434.31 \nLabel=Strip\t459\tX=19726.40\ty=-6358.36 \nLabel=Strip\t460\tX=20077.61\ty=-6278.21 \nLabel=Strip\t461\tX=19728.83\ty=-6202.39 \nLabel=Strip\t462\tX=20080.01\ty=-6122.11 \nLabel=Strip\t463\tX=19731.19\ty=-6046.42 \nLabel=Strip\t464\tX=20082.34\ty=-5966.01 \nLabel=Strip\t465\tX=19733.50\ty=-5890.45 \nLabel=Strip\t466\tX=20084.62\ty=-5809.90 \nLabel=Strip\t467\tX=19735.74\ty=-5734.48 \nLabel=Strip\t468\tX=20086.83\ty=-5653.79 \nLabel=Strip\t469\tX=19737.93\ty=-5578.51 \nLabel=Strip\t470\tX=20088.98\ty=-5497.68 \nLabel=Strip\t471\tX=19740.05\ty=-5422.53 \nLabel=Strip\t472\tX=20091.08\ty=-5341.57 \nLabel=Strip\t473\tX=19742.11\ty=-5266.55 \nLabel=Strip\t474\tX=20093.11\ty=-5185.46 \nLabel=Strip\t475\tX=19744.12\ty=-5110.57 \nLabel=Strip\t476\tX=20095.08\ty=-5029.34 \nLabel=Strip\t477\tX=19746.06\ty=-4954.59 \nLabel=Strip\t478\tX=20096.99\ty=-4873.22 \nLabel=Strip\t479\tX=19747.94\ty=-4798.60 \nLabel=Strip\t480\tX=20098.85\ty=-4717.10 \nLabel=Strip\t481\tX=19749.77\ty=-4642.62 \nLabel=Strip\t482\tX=20100.64\ty=-4560.98 \nLabel=Strip\t483\tX=19751.53\ty=-4486.63 \nLabel=Strip\t484\tX=20102.37\ty=-4404.85 \nLabel=Strip\t485\tX=19753.23\ty=-4330.64 \nLabel=Strip\t486\tX=20104.04\ty=-4248.73 \nLabel=Strip\t487\tX=19754.88\ty=-4174.65 \nLabel=Strip\t488\tX=20105.65\ty=-4092.60 \nLabel=Strip\t489\tX=19756.46\ty=-4018.65 \nLabel=Strip\t490\tX=20107.20\ty=-3936.47 \nLabel=Strip\t491\tX=19757.98\ty=-3862.65 \nLabel=Strip\t492\tX=20108.69\ty=-3780.33 \nLabel=Strip\t493\tX=19759.44\ty=-3706.66 \nLabel=Strip\t494\tX=20110.12\ty=-3624.20 \nLabel=Strip\t495\tX=19760.84\ty=-3550.66 \nLabel=Strip\t496\tX=20111.49\ty=-3468.06 \nLabel=Strip\t497\tX=19762.19\ty=-3394.66 \nLabel=Strip\t498\tX=20112.80\ty=-3311.93 \nLabel=Strip\t499\tX=19763.47\ty=-3238.65 \nLabel=Strip\t500\tX=20114.05\ty=-3155.79 \nLabel=Strip\t501\tX=19764.69\ty=-3082.65 \nLabel=Strip\t502\tX=20115.24\ty=-2999.64 \nLabel=Strip\t503\tX=19765.85\ty=-2926.64 \nLabel=Strip\t504\tX=20116.37\ty=-2843.50 \nLabel=Strip\t505\tX=19766.95\ty=-2770.63 \nLabel=Strip\t506\tX=20117.44\ty=-2687.36 \nLabel=Strip\t507\tX=19767.99\ty=-2614.62 \nLabel=Strip\t508\tX=20118.44\ty=-2531.21 \nLabel=Strip\t509\tX=19768.97\ty=-2458.61 \nLabel=Strip\t510\tX=20119.39\ty=-2375.06 \nLabel=Strip\t511\tX=19769.89\ty=-2302.59 \nLabel=Strip\t512\tX=20120.28\ty=-2218.91 \nLabel=Strip\t513\tX=19770.75\ty=-2146.58 \nLabel=Strip\t514\tX=20121.10\ty=-2062.76 \nLabel=Strip\t515\tX=19771.55\ty=-1990.56 \nLabel=Strip\t516\tX=20121.87\ty=-1906.60 \nLabel=Strip\t517\tX=19772.28\ty=-1834.54 \nLabel=Strip\t518\tX=20122.58\ty=-1750.45 \nLabel=Strip\t519\tX=19772.96\ty=-1678.52 \nLabel=Strip\t520\tX=20123.22\ty=-1594.29 \nLabel=Strip\t521\tX=19773.58\ty=-1522.50 \nLabel=Strip\t522\tX=20123.81\ty=-1438.13 \nLabel=Strip\t523\tX=19774.14\ty=-1366.47 \nLabel=Strip\t524\tX=20124.33\ty=-1281.98 \nLabel=Strip\t525\tX=19774.64\ty=-1210.45 \nLabel=Strip\t526\tX=20124.80\ty=-1125.81 \nLabel=Strip\t527\tX=19775.07\ty=-1054.42 \nLabel=Strip\t528\tX=20125.20\ty=-969.65 \nLabel=Strip\t529\tX=19775.45\ty=-898.39 \nLabel=Strip\t530\tX=20125.55\ty=-813.49 \nLabel=Strip\t531\tX=19775.77\ty=-742.36 \nLabel=Strip\t532\tX=20125.83\ty=-657.32 \nLabel=Strip\t533\tX=19776.02\ty=-586.33 \nLabel=Strip\t534\tX=20126.06\ty=-501.16 \nLabel=Strip\t535\tX=19776.22\ty=-430.30 \nLabel=Strip\t536\tX=20126.22\ty=-344.99 \nLabel=Strip\t537\tX=19776.36\ty=-274.26 \nLabel=Strip\t538\tX=20126.32\ty=-188.82 \nLabel=Strip\t539\tX=19776.43\ty=-118.23 \nLabel=Strip\t540\tX=20126.37\ty=-32.65 \nLabel=Strip\t541\tX=19776.45\ty=37.81 \nLabel=Strip\t542\tX=20126.35\ty=123.53 \nLabel=Strip\t543\tX=19776.40\ty=193.85 \nLabel=Strip\t544\tX=20126.27\ty=279.70 \nLabel=Strip\t545\tX=19776.30\ty=349.88 \nLabel=Strip\t546\tX=20126.13\ty=435.87 \nLabel=Strip\t547\tX=19776.13\ty=505.92 \nLabel=Strip\t548\tX=20125.93\ty=592.05 \nLabel=Strip\t549\tX=19775.91\ty=661.97 \nLabel=Strip\t550\tX=20125.68\ty=748.23 \nLabel=Strip\t551\tX=19775.62\ty=818.01 \nLabel=Strip\t552\tX=20125.36\ty=904.41 \nLabel=Strip\t553\tX=19775.28\ty=974.05 \nLabel=Strip\t554\tX=20124.98\ty=1060.59 \nLabel=Strip\t555\tX=19774.87\ty=1130.10 \nLabel=Strip\t556\tX=20124.54\ty=1216.77 \nLabel=Strip\t557\tX=19774.40\ty=1286.14 \nLabel=Strip\t558\tX=20124.04\ty=1372.95 \nLabel=Strip\t559\tX=19773.88\ty=1442.19 \nLabel=Strip\t560\tX=20123.48\ty=1529.13 \nLabel=Strip\t561\tX=19773.29\ty=1598.24 \nLabel=Strip\t562\tX=20122.86\ty=1685.32 \nLabel=Strip\t563\tX=19772.64\ty=1754.29 \nLabel=Strip\t564\tX=20122.17\ty=1841.50 \nLabel=Strip\t565\tX=19771.93\ty=1910.34 \nLabel=Strip\t566\tX=20121.43\ty=1997.69 \nLabel=Strip\t567\tX=19771.17\ty=2066.39 \nLabel=Strip\t568\tX=20120.63\ty=2153.88 \nLabel=Strip\t569\tX=19770.34\ty=2222.44 \nLabel=Strip\t570\tX=20119.77\ty=2310.06 \nLabel=Strip\t571\tX=19769.45\ty=2378.50 \nLabel=Strip\t572\tX=20118.85\ty=2466.25 \nLabel=Strip\t573\tX=19768.50\ty=2534.55 \nLabel=Strip\t574\tX=20117.86\ty=2622.44 \nLabel=Strip\t575\tX=19767.49\ty=2690.61 \nLabel=Strip\t576\tX=20116.82\ty=2778.63 \nLabel=Strip\t577\tX=19766.42\ty=2846.67 \nLabel=Strip\t578\tX=20115.72\ty=2934.83 \nLabel=Strip\t579\tX=19765.29\ty=3002.72 \nLabel=Strip\t580\tX=20114.55\ty=3091.02 \nLabel=Strip\t581\tX=19764.10\ty=3158.78 \nLabel=Strip\t582\tX=20113.33\ty=3247.21 \nLabel=Strip\t583\tX=19762.85\ty=3314.84 \nLabel=Strip\t584\tX=20112.04\ty=3403.41 \nLabel=Strip\t585\tX=19761.54\ty=3470.90 \nLabel=Strip\t586\tX=20110.70\ty=3559.60 \nLabel=Strip\t587\tX=19760.17\ty=3626.96 \nLabel=Strip\t588\tX=20109.29\ty=3715.80 \nLabel=Strip\t589\tX=19758.74\ty=3783.02 \nLabel=Strip\t590\tX=20107.83\ty=3872.00 \nLabel=Strip\t591\tX=19757.24\ty=3939.08 \nLabel=Strip\t592\tX=20106.30\ty=4028.19 \nLabel=Strip\t593\tX=19755.69\ty=4095.15 \nLabel=Strip\t594\tX=20104.71\ty=4184.39 \nLabel=Strip\t595\tX=19754.08\ty=4251.21 \nLabel=Strip\t596\tX=20103.07\ty=4340.59 \nLabel=Strip\t597\tX=19752.41\ty=4407.27 \nLabel=Strip\t598\tX=20101.36\ty=4496.79 \nLabel=Strip\t599\tX=19750.67\ty=4563.34 \nLabel=Strip\t600\tX=20099.59\ty=4652.99 \nLabel=Strip\t601\tX=19748.88\ty=4719.40 \nLabel=Strip\t602\tX=20097.76\ty=4809.19 \nLabel=Strip\t603\tX=19747.03\ty=4875.47 \nLabel=Strip\t604\tX=20095.87\ty=4965.39 \nLabel=Strip\t605\tX=19745.11\ty=5031.54 \nLabel=Strip\t606\tX=20093.93\ty=5121.59 \nLabel=Strip\t607\tX=19743.14\ty=5187.60 \nLabel=Strip\t608\tX=20091.92\ty=5277.80 \nLabel=Strip\t609\tX=19741.10\ty=5343.67 \nLabel=Strip\t610\tX=20089.85\ty=5434.00 \nLabel=Strip\t611\tX=19739.01\ty=5499.74 \nLabel=Strip\t612\tX=20087.72\ty=5590.20 \nLabel=Strip\t613\tX=19736.85\ty=5655.81 \nLabel=Strip\t614\tX=20085.53\ty=5746.41 \nLabel=Strip\t615\tX=19734.64\ty=5811.88 \nLabel=Strip\t616\tX=20083.28\ty=5902.61 \nLabel=Strip\t617\tX=19732.36\ty=5967.95 \nLabel=Strip\t618\tX=20080.97\ty=6058.82 \nLabel=Strip\t619\tX=19730.03\ty=6124.02 \nLabel=Strip\t620\tX=20078.59\ty=6215.02 \nLabel=Strip\t621\tX=19727.63\ty=6280.09 \nLabel=Strip\t622\tX=20076.16\ty=6371.23 \nLabel=Strip\t623\tX=19725.17\ty=6436.16 \nLabel=Strip\t624\tX=20073.67\ty=6527.43 \nLabel=Strip\t625\tX=19722.65\ty=6592.23 \nLabel=Strip\t626\tX=20071.12\ty=6683.64 \nLabel=Strip\t627\tX=19720.08\ty=6748.30 \nLabel=Strip\t628\tX=20068.50\ty=6839.85 \nLabel=Strip\t629\tX=19717.44\ty=6904.37 \nLabel=Strip\t630\tX=20065.83\ty=6996.06 \nLabel=Strip\t631\tX=19714.74\ty=7060.45 \nLabel=Strip\t632\tX=20063.10\ty=7152.26 \nLabel=Strip\t633\tX=19711.98\ty=7216.52 \nLabel=Strip\t634\tX=20060.30\ty=7308.47 \nLabel=Strip\t635\tX=19709.16\ty=7372.59 \nLabel=Strip\t636\tX=20057.45\ty=7464.68 \nLabel=Strip\t637\tX=19706.28\ty=7528.66 \nLabel=Strip\t638\tX=20054.53\ty=7620.89 \nLabel=Strip\t639\tX=19703.34\ty=7684.74 \nLabel=Strip\t640\tX=20051.56\ty=7777.09 \nLabel=Strip\t641\tX=19700.34\ty=7840.81 \nLabel=Strip\t642\tX=20048.52\ty=7933.30 \nLabel=Strip\t643\tX=19697.28\ty=7996.88 \nLabel=Strip\t644\tX=20045.43\ty=8089.51 \nLabel=Strip\t645\tX=19694.16\ty=8152.96 \nLabel=Strip\t646\tX=20042.27\ty=8245.72 \nLabel=Strip\t647\tX=19690.98\ty=8309.03 \nLabel=Strip\t648\tX=20039.05\ty=8401.93 \nLabel=Strip\t649\tX=19687.74\ty=8465.10 \nLabel=Strip\t650\tX=20035.78\ty=8558.14 \nLabel=Strip\t651\tX=19684.44\ty=8621.18 \nLabel=Strip\t652\tX=20032.44\ty=8714.34 \nLabel=Strip\t653\tX=19681.08\ty=8777.25 \nLabel=Strip\t654\tX=20029.04\ty=8870.55 \nLabel=Strip\t655\tX=19677.65\ty=8933.32 \nLabel=Strip\t656\tX=20025.58\ty=9026.76 \nLabel=Strip\t657\tX=19674.17\ty=9089.40 \nLabel=Strip\t658\tX=20022.06\ty=9182.97 \nLabel=Strip\t659\tX=19670.63\ty=9245.47 \nLabel=Strip\t660\tX=20018.48\ty=9339.18 \nLabel=Strip\t661\tX=19667.03\ty=9401.54 \nLabel=Strip\t662\tX=20014.84\ty=9495.39 \nLabel=Strip\t663\tX=19663.36\ty=9557.62 \nLabel=Strip\t664\tX=20011.14\ty=9651.60 \nLabel=Strip\t665\tX=19659.64\ty=9713.69 \nLabel=Strip\t666\tX=20007.38\ty=9807.80 \nLabel=Strip\t667\tX=19655.85\ty=9869.76 \nLabel=Strip\t668\tX=20003.56\ty=9964.01 \nLabel=Strip\t669\tX=19652.01\ty=10025.84 \nLabel=Strip\t670\tX=19999.68\ty=10120.22 \nLabel=Strip\t671\tX=19648.10\ty=10181.91 \nLabel=Strip\t672\tX=19995.74\ty=10276.43 \nLabel=Strip\t673\tX=19644.14\ty=10337.98 \nLabel=Strip\t674\tX=19991.74\ty=10432.63 \nLabel=Strip\t675\tX=19640.11\ty=10494.05 \nLabel=Strip\t676\tX=19987.67\ty=10588.84 \nLabel=Strip\t677\tX=19636.02\ty=10650.13 \nLabel=Strip\t678\tX=19983.55\ty=10745.05 \nLabel=Strip\t679\tX=19631.88\ty=10806.20 \nLabel=Strip\t680\tX=19979.37\ty=10901.25 \nLabel=Strip\t681\tX=19627.67\ty=10962.27 \nLabel=Strip\t682\tX=19975.12\ty=11057.46 \nLabel=Strip\t683\tX=19623.40\ty=11118.34 \nLabel=Strip\t684\tX=19970.82\ty=11213.67 \nLabel=Strip\t685\tX=19619.08\ty=11274.41 \nLabel=Strip\t686\tX=19966.46\ty=11369.87 \nLabel=Strip\t687\tX=19614.69\ty=11430.48 \nLabel=Strip\t688\tX=19962.03\ty=11526.08 \nLabel=Strip\t689\tX=19610.24\ty=11586.55 \nLabel=Strip\t690\tX=19957.55\ty=11682.28 \nLabel=Strip\t691\tX=19605.73\ty=11742.62 \nLabel=Strip\t692\tX=19953.00\ty=11838.49 \nLabel=Strip\t693\tX=19601.16\ty=11898.69 \nLabel=Strip\t694\tX=19948.39\ty=11994.69 \nLabel=Strip\t695\tX=19596.53\ty=12054.76 \nLabel=Strip\t696\tX=19943.73\ty=12150.89 \nLabel=Strip\t697\tX=19591.84\ty=12210.83 \nLabel=Strip\t698\tX=19939.00\ty=12307.10 \nLabel=Strip\t699\tX=19587.09\ty=12366.90 \nLabel=Strip\t700\tX=19934.21\ty=12463.30 \nLabel=Strip\t701\tX=19582.28\ty=12522.96 \nLabel=Strip\t702\tX=19929.36\ty=12619.50 \nLabel=Strip\t703\tX=19577.41\ty=12679.03 \nLabel=Strip\t704\tX=19924.46\ty=12775.70 \nLabel=Strip\t705\tX=19572.48\ty=12835.09 \nLabel=Strip\t706\tX=19919.49\ty=12931.90 \nLabel=Strip\t707\tX=19567.49\ty=12991.16 \nLabel=Strip\t708\tX=19914.46\ty=13088.10 \nLabel=Strip\t709\tX=19562.44\ty=13147.22 \nLabel=Strip\t710\tX=19909.37\ty=13244.30 \nLabel=Strip\t711\tX=19557.32\ty=13303.29 \nLabel=Strip\t712\tX=19904.22\ty=13400.50 \nLabel=Strip\t713\tX=19552.15\ty=13459.35 \nLabel=Strip\t714\tX=19899.01\ty=13556.70 \nLabel=Strip\t715\tX=19546.92\ty=13615.41 \nLabel=Strip\t716\tX=19893.74\ty=13712.90 \nLabel=Strip\t717\tX=19541.62\ty=13771.48 \nLabel=Strip\t718\tX=19888.41\ty=13869.09 \nLabel=Strip\t719\tX=19536.27\ty=13927.54 \nLabel=Strip\t720\tX=19883.01\ty=14025.29 \nLabel=Strip\t721\tX=19530.85\ty=14083.60 \nLabel=Strip\t722\tX=19877.56\ty=14181.48 \nLabel=Strip\t723\tX=19525.38\ty=14239.66 \nLabel=Strip\t724\tX=19872.05\ty=14337.68 \nLabel=Strip\t725\tX=19519.84\ty=14395.72 \nLabel=Strip\t726\tX=19866.48\ty=14493.87 \nLabel=Strip\t727\tX=19514.25\ty=14551.77 \nLabel=Strip\t728\tX=19860.84\ty=14650.06 \nLabel=Strip\t729\tX=19508.59\ty=14707.83 \nLabel=Strip\t730\tX=19855.15\ty=14806.25 \nLabel=Strip\t731\tX=19502.88\ty=14863.89 \nLabel=Strip\t732\tX=19849.39\ty=14962.44 \nLabel=Strip\t733\tX=19497.10\ty=15019.96 \nLabel=Strip\t734\tX=19843.58\ty=15118.63 \nLabel=Strip\t735\tX=19491.26\ty=15176.00 \nLabel=Strip\t736\tX=19837.70\ty=15274.82 \nLabel=Strip\t737\tX=19485.37\ty=15332.05 \nLabel=Strip\t738\tX=19831.77\ty=15431.01 \nLabel=Strip\t739\tX=19479.41\ty=15488.10 \nLabel=Strip\t740\tX=19825.77\ty=15587.20 \nLabel=Strip\t741\tX=19473.39\ty=15644.15 \nLabel=Strip\t742\tX=19819.72\ty=15743.38 \nLabel=Strip\t743\tX=19467.31\ty=15800.20 \nLabel=Strip\t744\tX=19813.60\ty=15899.57 \nLabel=Strip\t745\tX=19461.17\ty=15956.25 \nLabel=Strip\t746\tX=19807.42\ty=16055.75 \nLabel=Strip\t747\tX=19454.97\ty=16112.30 \nLabel=Strip\t748\tX=19801.18\ty=16211.93 \nLabel=Strip\t749\tX=19448.71\ty=16268.35 \nLabel=Strip\t750\tX=19794.88\ty=16368.11 \nLabel=Strip\t751\tX=19442.39\ty=16424.39 \nLabel=Strip\t752\tX=19788.53\ty=16524.30 \nLabel=Strip\t753\tX=19436.01\ty=16580.44 \nLabel=Strip\t754\tX=19782.11\ty=16680.47 \nLabel=Strip\t755\tX=19429.57\ty=16736.48 \nLabel=Strip\t756\tX=19775.63\ty=16836.65 \nLabel=Strip\t757\tX=19423.07\ty=16892.52 \nLabel=Strip\t758\tX=19769.09\ty=16992.83 \nLabel=Strip\t759\tX=19416.51\ty=17048.57 \nLabel=Strip\t760\tX=19762.49\ty=17149.00 \nLabel=Strip\t761\tX=19409.89\ty=17204.61 \nLabel=Strip\t762\tX=19755.83\ty=17305.18 
